vi "oax_Open File.vi"(8 "error in":errorcluster) -> (0 "error out":errorcluster, 1 "Vibration File Path (.wav)":path, 2 "Tacho File Path (.wav)":path, 3 "File Path (.dat)":path=path "C:/Program Files/National Instruments/LabVIEW 8.2/examples/Order Analysis/Example Data/1x_2x_10x(run up and down).dat", 4 "Tacho info out":T1={"pulse / rev"=1, "threshold (auto)"=inf, "slope (Rising)"=0} {"slope (Rising)" items=["Rising", "Falling"]}, 5 "Enum":enum16{"Load .wav file", "Load .dat file"}(ring)=enum."Load .dat file", 7 "OK?":bool=TRUE)   [LabVIEW 2017]
panel:
  in  "File Type":u16(ring) items=["wav", "dat"]
  in  "Path tab":enum32{"Load .wav", "Load .dat"}(tab)=enum."Load .dat"
  in  "Vibration File Path (.wav)":path
  in  "Tacho File Path (.wav)":path
  in  "Tacho info":T2={"Pulse / Rev"=1, "Threshold (Auto)"=inf, "Slope (Rising)"=0} {"Slope (Rising)" items=["Rising", "Falling"]}
  in  "File Path (.dat)":path
  in  "Cancel":bool
  in  "OK":bool
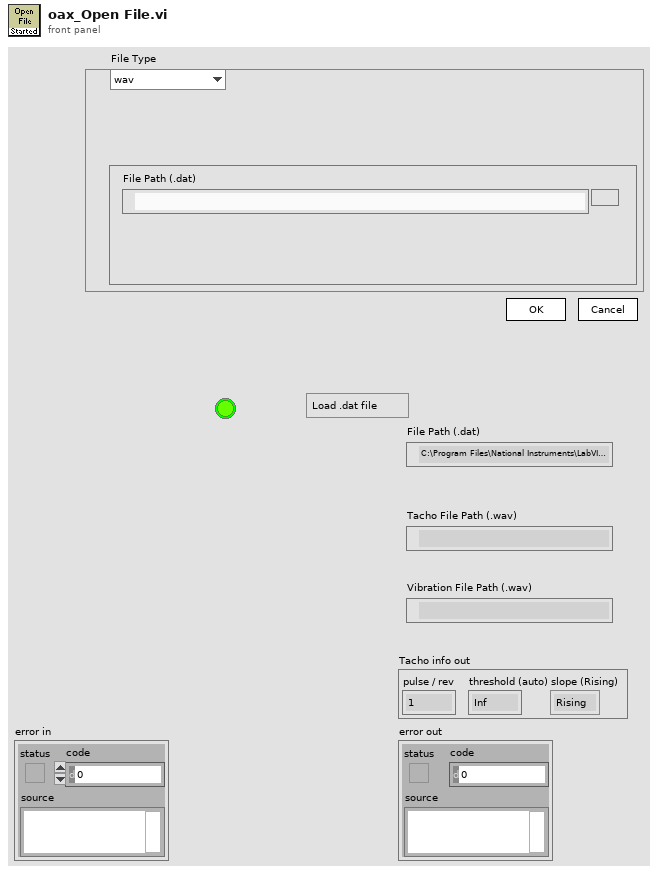
[diagram p1: front panel]
types:
  T1 = cluster{"pulse / rev":i32, "threshold (auto)":dbl, "slope (Rising)":u16}
  T2 = cluster{"Pulse / Rev":i32, "Threshold (Auto)":dbl, "Slope (Rising)":u16}
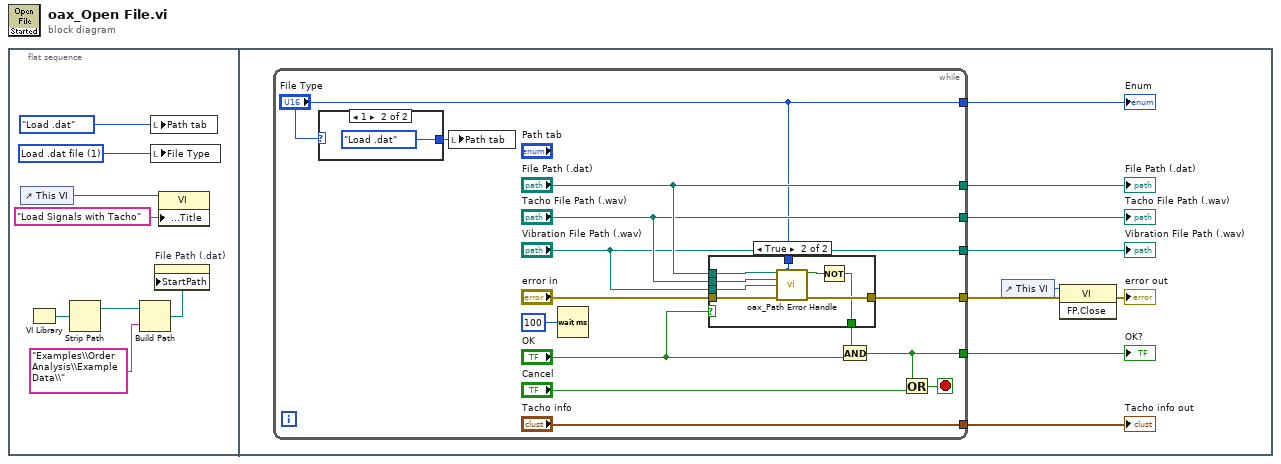
[diagram p0: block diagram]
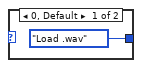
[diagram p2: hidden frame]
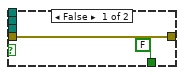
[diagram p3: hidden frame]
diagram:
  n1 = flat-sequence {
    frame #0 {
      w7 = u16 1 items=["Load .wav file", "Load .dat file"] ("File Type")
      n2 = control-ref of="This VI"() -> (w5:refnum<vi>)
      n3 = VI Library() -> (path=w4:path)
      n4 = Strip Path(path=w4) -> (stripped path=w3:path)  [unwired: 1 out]
      n5 = Build Path(base path=w3, name or relative path="Examples\\Order Analysis\\Example Data\\" ("relative path")) -> (appended path=w1:path)
      n6 = local write "Path tab"(enum32{"Load .wav", "Load .dat"}."Load .dat" ("Path tab")) -> ()
      n7 = local write "File Type"(w7) -> ()
      n8 = property on="File Path (.dat)" class="Path"("StartPath"=w1) -> ()  [unwired: 2 in, 2 out]
      n9 = property class="VI"(reference=w5, "Front Panel.Title"="Load Signals with Tacho" ("Front Panel Window:Title")) -> ()  [unwired: 1 in, 2 out]
    }
    frame #1 {
      n10 = while {
        tunnel: ["File Type"] -> w17
        tunnel: ["File Path (.dat)"] -> w16
        tunnel: ["Tacho File Path (.wav)"] -> w15
        tunnel: ["Vibration File Path (.wav)"] -> w14
        tunnel: [w22] -> w13
        tunnel: [w24] -> w12
        tunnel: ["Tacho info"] -> w11
        stop <- w28 stop-if-true
        n11 = case shown="1" "File Type" {
          tunnel: [enum32{"Load .wav", "Load .dat"}."Load .wav" ("Path tab") enum32{"Load .wav", "Load .dat"}."Load .dat" ("Path tab")] -> w19
          frame 0, Default {
          }
          frame 1 {
          }
        }
        n12 = local write "Path tab"(w19) -> ()
        n13 = Wait (ms)(milliseconds to wait=u32 100) -> ()  [unwired: 1 out]
        n14 = case shown="True" "OK" {
          tunnel: "File Type" -> [_ w43]
          tunnel: "error in" -> [w35 w42]
          tunnel: "File Path (.dat)" -> [_ w40]
          tunnel: "Tacho File Path (.wav)" -> [_ w39]
          tunnel: "Vibration File Path (.wav)" -> [_ w38]
          tunnel: [w35 w37] -> w24
          tunnel: [FALSE w36] -> w21
          frame False {
          }
          frame True {
            n15 = call <vilib>:"oax_Path Error Handle.vi"("File Path (.dat)"=w40, "Ring"=w43, "Tacho File Path (.wav)"=w39, "Vibration File Path (.wav)"=w38, "error In"=w42) -> ("Error"=w41:bool, "error Out"=w37:errorcluster)  [unwired: 9 in]
            n16 = Not(x=w41) -> (.not. x?=w36:bool)
          }
        }
        n17 = And(x=w21, y="OK") -> (x .and. y?=w22:bool)
        n18 = Or(x=w22, y="Cancel") -> (x .or. y?=w28:bool)
      }
      "Enum" <- w17
      "Tacho File Path (.wav)" <- w15
      "File Path (.dat)" <- w16
      "Vibration File Path (.wav)" <- w14
      "Tacho info out" <- w11
      "OK?" <- w13
      n19 = control-ref of="This VI"() -> (w10:refnum<vi>)
      n20 = invoke class="VI" method="FP.Close"(reference=w10, error in=w12) -> (error out=→"error out":errorcluster)  [unwired: 1 in, 2 out]
    }
  }
